vi "DSCMonitoring_p.vi"(0 "MoAgSy_Host":refnum<class "MoAgSy_Host.lvclass">, 2 "msTimeout (-1)":i32=-1, 5 "error in (no error)":errorcluster) -> (9 "nofTasksWaiting":i32, 11 "nofThreads":i32, 13 "initialNofThreads":i32, 14 "dup MoAgSy_Host":refnum<class "MoAgSy_Host.lvclass">, 15 "Host timed out?":bool, 16 "Registration Array":T1(array[cluster]), 17 "Agent timed out?":bool, 18 "Reg Array":T1(array[cluster]), 19 "error out":errorcluster)   [LabVIEW 2009, in "MoAgSy.lvlib" / "MoAgSy_Host.lvclass"]
uses:
  MoAgSy_Host.lvclass
  HGF_BaseClasses/HGF_NetworkVisitor/HGF_NetworkVisitor.lvclass
  HGF_BaseClasses/HGF_TriggeredEvent/HGF_TriggeredEvent.lvclass
  MoAgSy_Host.lvclass/MoAgSy_Host.ctl
  HGF_BaseClasses/HGF_ThreadTask/HGF_ThreadTask.lvclass
  HGF_BaseClasses/HGF_ThreadPool/HGF_ThreadPool.lvclass
  HGF_BaseClasses/HGF_Reference/HGF_Reference.lvclass
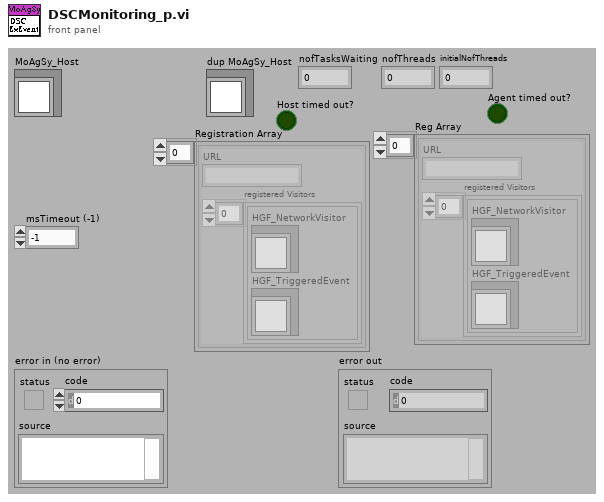
[diagram p1: front panel]
types:
  T1 = cluster{"URL":string, "registered Visitors":cluster{"HGF_NetworkVisitor":refnum<class "HGF_NetworkVisitor.lvclass">, "HGF_TriggeredEvent":refnum<class "HGF_TriggeredEvent.lvclass">}[]}[]
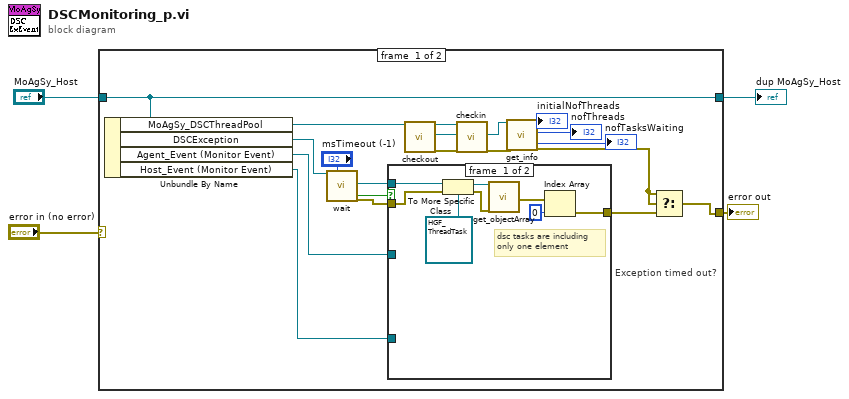
[diagram p0: block diagram]
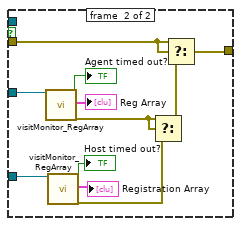
[diagram p2: hidden frame]
diagram:
  n1 = case shown="No Error" "error in (no error)" {
    selector: "error in (no error)" -> [_ w44]
    tunnel: "MoAgSy_Host" -> [w23 w43]
    tunnel: [w23 w43] -> w2
    tunnel: [w10 w44] -> w1
    frame #0 {
      n2 = Unbundle By Name(w23) -> ("MoAgSy_DSCThreadPool"=w15:refnum<class "HGF_Reference.lvclass">, "DSCException"=w22:refnum<class "HGF_TriggeredEvent.lvclass">, "Agent_Event (Monitor Event)"=w17:refnum<class "HGF_Event.lvclass">, "Host_Event (Monitor Event)"=w16:refnum<class "HGF_Event.lvclass">)
      n3 = call-dynamic "wait.vi"("HGF_Event"=w22, "msTimeout (-1)"="msTimeout (-1)") -> ("Object"=w21:refnum<class>, "timed out"=w19:bool, "error out"=w20:errorcluster)  [unwired: 14 in, 1 out]
      n4 = case "Exception timed out?" shown="True" w19 {
        tunnel: w21 -> [w31 _]
        tunnel: w20 -> [w30 w41]
        tunnel: [w24 w40] -> w9
        tunnel: w17 -> [_ w42]
        tunnel: w16 -> [_ w34]
        frame #0 {
          # "dsc tasks are including\nonly one element"
          n5 = To More Specific Class(target class=refnum<class "HGF_ThreadTask.lvclass"> refnum ("HGF_BaseClasses.lvlib:HGF_ThreadTask.lvclass"), reference=w31, error in=w30) -> (specific class reference=w28:refnum<class "HGF_ThreadTask.lvclass">, error out=w27:errorcluster)
          n6 = call "get_objectArray.vi"("HGF_ThreadTask"=w28, "error in (no error)"=w27) -> ("errorArray"=w26:errorcluster[])  [unwired: 14 in, 3 out]
          n7 = Index Array(array=w26, index=0) -> (element=w24:errorcluster)
        }
        frame #1 {
          n8 = call "visitMonitor_RegArray.vi"("HGF_Event"=w42) -> ("timed out?"=→"Agent timed out?":bool, "Registration Array"=→"Reg Array":T1, "error out"=w38:errorcluster)  [unwired: 16 in]
          n9 = call "visitMonitor_RegArray.vi"("HGF_Event"=w34) -> ("timed out?"=→"Host timed out?":bool, "Registration Array"=→"Registration Array":T1, "error out"=w36:errorcluster)  [unwired: 16 in]
          n10 = Select(t=w38, s=w38, f=w36) -> (s? t:f=w37:errorcluster)
          n11 = Select(t=w41, s=w41, f=w37) -> (s? t:f=w40:errorcluster)
        }
      }
      n12 = call "checkout.vi"("HGF_ThreadPool_Reference"=w15) -> ("dup HGF_ThreadPool_Reference"=w13:refnum<class "HGF_Reference.lvclass">, "HGF_ThreadPool"=w14:refnum<class "HGF_ThreadPool.lvclass">, "error out"=w12:errorcluster)  [unwired: 15 in, 1 out]
      n13 = call "checkin.vi"("HGF_Reference"=w13, "Object"=w14, "error in (no error)"=w12) -> ("error out"=w11:errorcluster)  [unwired: 14 in, 2 out]
      n14 = call "get_info.vi"("HGF_ThreadPool"=w14, "error in (no error)"=w11) -> ("nofTasksWaiting"=→"nofTasksWaiting":i32, "initialNofThreads"=→"initialNofThreads":i32, "nofThreads"=→"nofThreads":i32, "error out"=w8:errorcluster)  [unwired: 8 in, 6 out]
      n15 = Select(t=w8, s=w8, f=w9) -> (s? t:f=w10:errorcluster)
    }
    frame #1 {
    }
  }
  "error out" <- w1
  "dup MoAgSy_Host" <- w2
